vi "FinalProjMeasureRMSJ&J.vi"() -> (2 "Waveform Graph":dynamicdata(graph))   [LabVIEW 2015]
uses:
  <vilib>/ptbypt/NI_PtbyPt.lvlib
panel:
  out "Frequency":cluster{"all rows":dbl[], "all rows":dbl[]}(graph)
  in  "file path (use dialog)":path
  in  "Peak Detector":T1 {"threshold valley" format="%0.2f"; "threshold peak" format="%0.2f"}
  in  "Waveform Controls":T2
  out "Acceleration":cluster{"all rows":dbl[], "all rows":dbl[]}(graph)
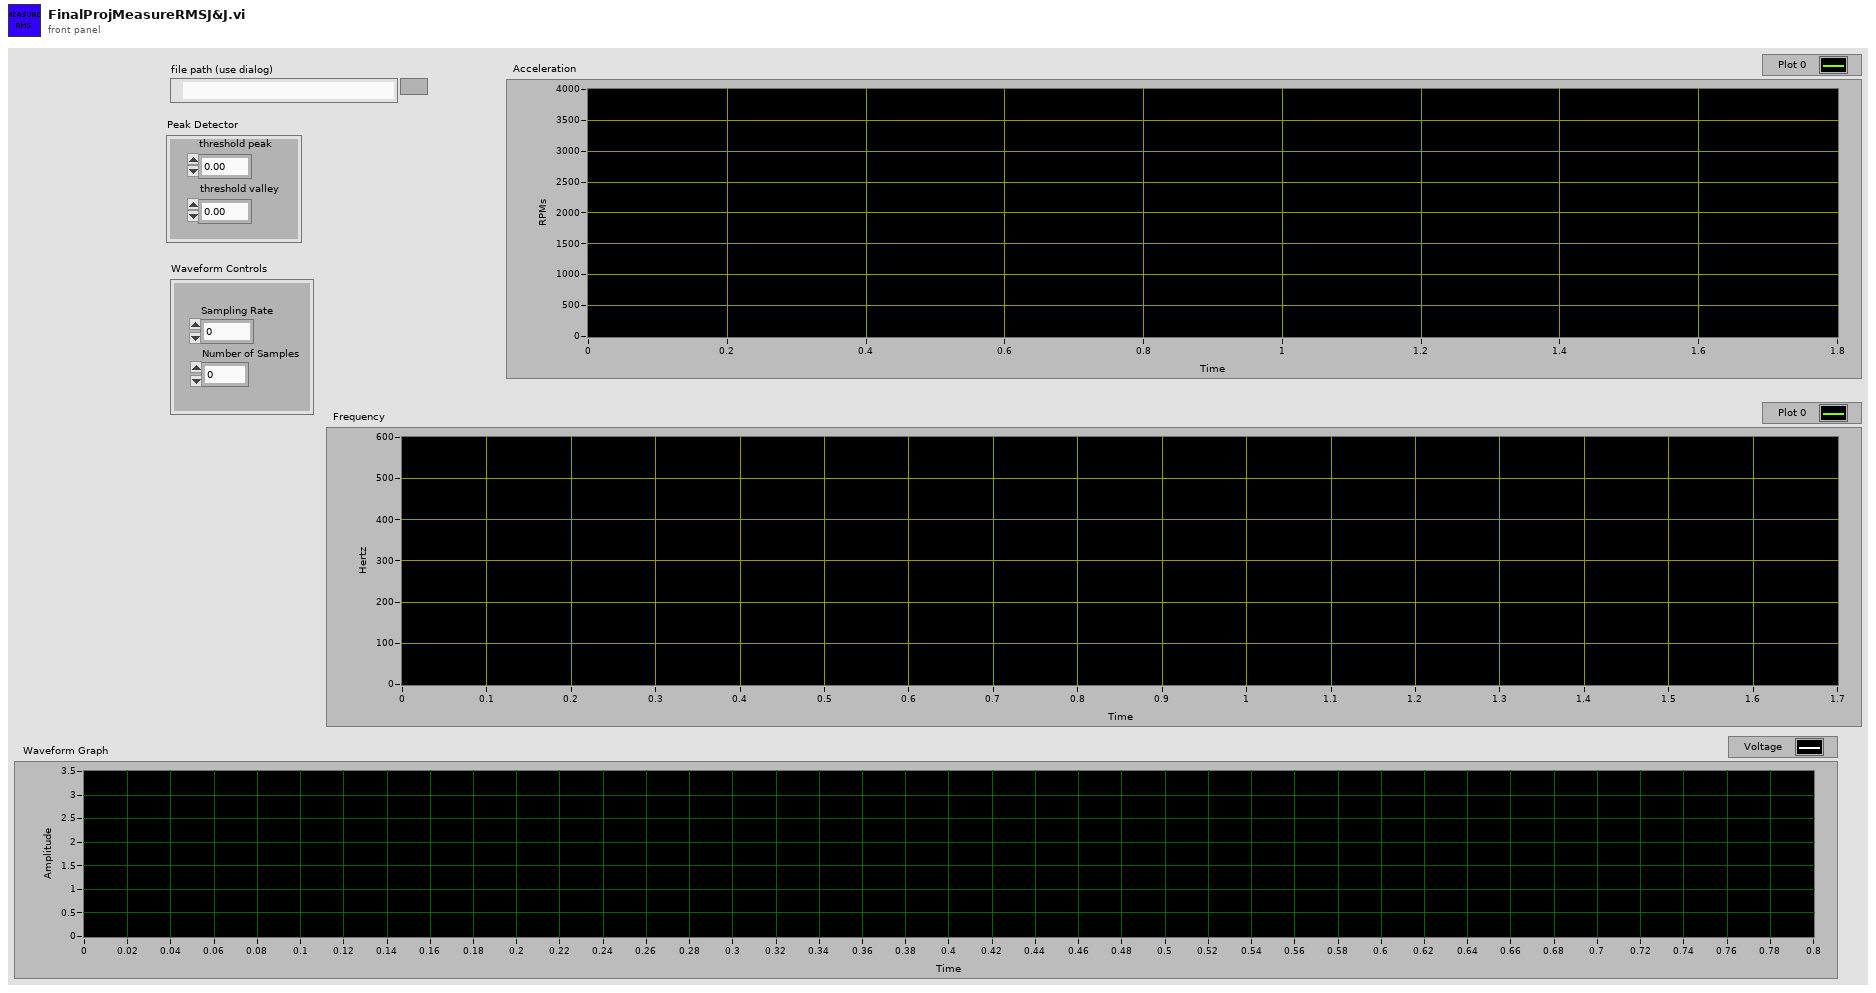
[diagram p1: front panel]
types:
  T1 = cluster{"threshold peak":dbl, "threshold valley":dbl}
  T2 = cluster{"Sampling Rate":dbl, "Number of Samples":dbl}
  T3 = enum16{"open", "replace", "create", "open or create", "replace or create", "replace or create with confirmation"}
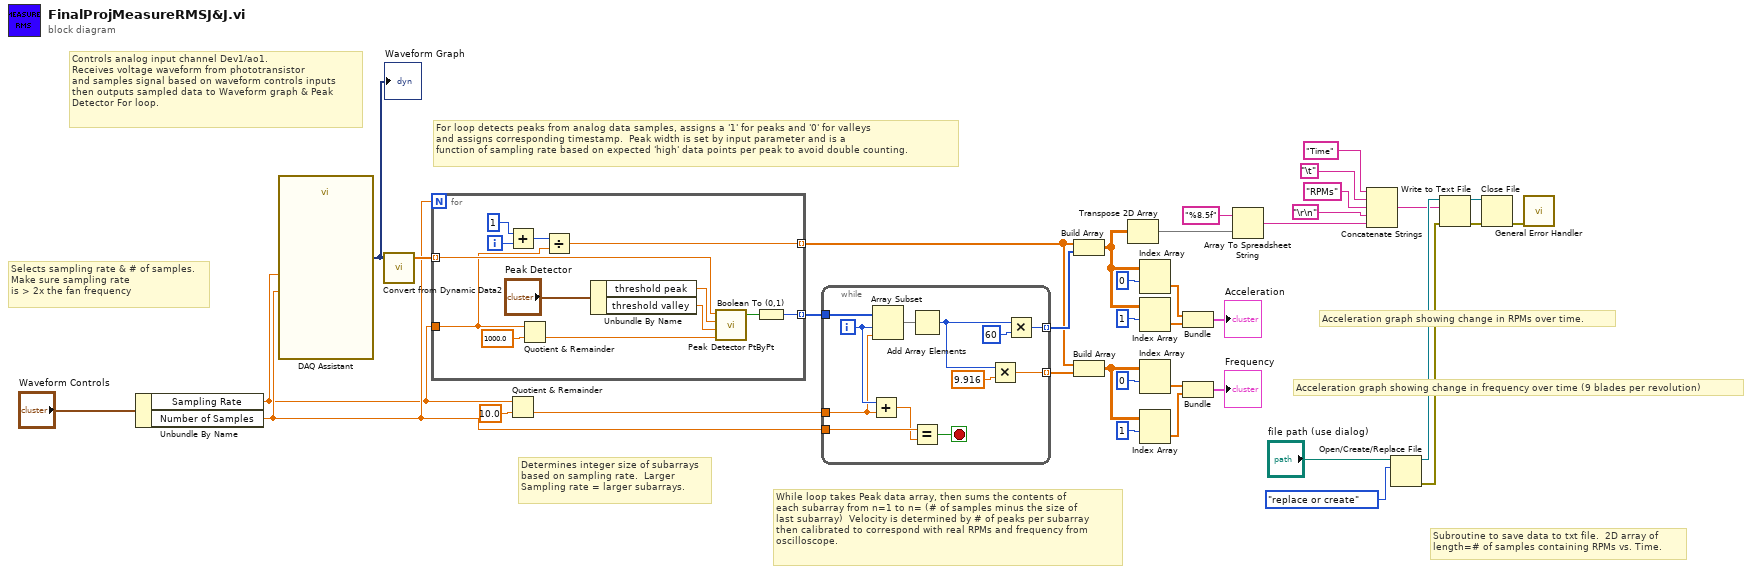
[diagram p0: block diagram]
diagram:
  # "Acceleration graph showing change in frequency over time (9 blades per revolution)"
  # "Acceleration graph showing change in RPMs over time."
  # "Subroutine to save data to txt file.  2D array of \nlength=# of samples containing RPMs vs. Time."
  # "While loop takes Peak data array, then sums the contents of\neach subarray from n=1 to n= (# of samples minus the size of \nlast subarray)  Velocity is determined by # of peaks per subarray\nthen calibrated to correspond with real RPMs and frequency from\noscilloscope."
  # "For loop detects peaks from analog data samples, assigns a '1' for peaks and '0' for valleys\nand assigns corresponding timestamp.  Peak width is set by input parameter and is a\nfunction of sampling rate based on expected 'high' data points per peak to avoid double counting."
  # "Determines integer size of subarrays\nbased on sampling rate.  Larger\nSampling rate = larger subarrays."
  # "Controls analog input channel Dev1/ao1.\nReceives voltage waveform from phototransistor\nand samples signal based on waveform controls inputs\nthen outputs sampled data to Waveform graph & Peak\nDetector For loop."
  # "Selects sampling rate & # of samples.\nMake sure sampling rate \nis > 2x the fan frequency"
  n1 = Unbundle By Name("Waveform Controls") -> ("Sampling Rate"=w10:dbl, "Number of Samples"=w11:dbl)
  n2 = call "DAQ Assistant"("rate"=w10, "number of samples"=w11) -> ("data"=w25:dynamicdata)  [unwired: 15 in, 2 out]
  "Waveform Graph" <- w25
  n3 = call "Convert from Dynamic Data2"("Dynamic Data Type"=w25) -> ("Array"=w23:dbl[])  [unwired: 3 in]
  n4 = for {
    N: w11 -> [_]
    tunnel: w10 -> [w41]
    tunnel: [w48] -> w3 mode=indexing
    tunnel: w23 -> [w47] mode=indexing
    tunnel: [w45] -> w22 mode=indexing
    i -> [w51]
    n5 = Add(x=1, y=w51) -> (x+y=w49:i32)
    n6 = Quotient & Remainder(x=w41, y=1000.0) -> (floor(x/y)=w39:dbl)  [unwired: 1 out]
    n7 = Divide(x=w49, y=w41) -> (x/y=w48:dbl)
    n8 = Unbundle By Name("Peak Detector") -> ("threshold peak"=w43:dbl, "threshold valley"=w42:dbl)
    n9 = call <vilib>:"Peak Detector PtByPt.vi"("x"=w47, "threshold peak"=w43, "threshold valley"=w42, "width"=w39) -> ("peak"=w46:bool)  [unwired: 1 in, 2 out]
    n10 = Boolean To (0,1)(Boolean=w46) -> (0, 1=w45:i16)
  }
  n11 = Quotient & Remainder(x=w10, y=10.0) -> (floor(x/y)=w19:dbl)  [unwired: 1 out]
  n12 = while {
    tunnel: w22 -> [w63]
    tunnel: [w59] -> w21 mode=indexing
    tunnel: w11 -> [w61]
    tunnel: w19 -> [w56]
    tunnel: [w52] -> w1 mode=indexing
    i -> [w57]
    stop <- w60 stop-if-true
    n13 = Add(x=w57, y=w56) -> (x+y=w55:dbl)
    n14 = Array Subset(array=w63, index=w57, length=w56) -> (w62:i16[])
    n15 = Add Array Elements(numeric array=w62) -> (sum=w53:i16)
    n16 = Equal?(x=w61, y=w55) -> (x = y?=w60:bool)
    n17 = Multiply(x=w53, y=9.916) -> (x*y=w52:dbl)
    n18 = Multiply(x=w53, y=60) -> (x*y=w59:i32)
  }
  n19 = Build Array(w3, w21) -> (w13:dbl[][])
  n20 = Build Array(w3, w1) -> (w2:dbl[][])
  n21 = Transpose 2D Array(2D array=w13) -> (transposed array=w24:dbl[][])
  n22 = Index Array(array=w13, index (row)=0 ("index")) -> (element=w16:dbl[])  [unwired: 1 in]
  n23 = Index Array(array=w13, index (row)=1 ("index")) -> (element=w15:dbl[])  [unwired: 1 in]
  n24 = Index Array(array=w2, index (row)=0 ("index")) -> (element=w6:dbl[])  [unwired: 1 in]
  n25 = Index Array(array=w2, index (row)=1 ("index")) -> (element=w5:dbl[])  [unwired: 1 in]
  n26 = Bundle(w16, w15) -> (→"Acceleration":cluster{dbl[], dbl[]})  [unwired: 1 in]
  n27 = Bundle(w6, w5) -> (→"Frequency":cluster{dbl[], dbl[]})  [unwired: 1 in]
  n28 = Array To Spreadsheet String(array=w24, 3:"%8.5f" ("format string")) -> (spreadsheet string=w27:string)  [unwired: 1 in]
  n29 = Concatenate Strings("Time" ("string"), "\t", "RPMs" ("string"), "\r\n", w27) -> (w26:string)
  n30 = Open/Create/Replace File(file path (use dialog)="file path (use dialog)", operation (0:open)=T3."replace or create") -> (refnum out=w35:refnum<file>, error out=w36:errorcluster)  [unwired: 4 in, 1 out]
  n31 = Write to Text File(file (use dialog)=w35, text=w26, error in=w36) -> (refnum out=w34:refnum<file>, error out=w37:errorcluster)  [unwired: 1 in, 1 out]
  n32 = Close File(refnum=w34, error in=w37) -> (error out=w38:errorcluster)  [unwired: 1 out]
  n33 = call <vilib>:"General Error Handler.vi"("error in (no error)"=w38) -> ()  [unwired: 10 in, 5 out]
